vi "PauseSong.vi"(8 "error in (no error)":errorcluster, 10 "Message Queues in":T1, 11 "UI Refs in":T2) -> (0 "error out":errorcluster, 2 "Message Queues out":T1, 3 "UI Refs out":T2)   [LabVIEW 2015]
uses:
  Controls & Type Defs/UI Data.ctl
  support/Message Queue/All Message Queues.ctl
  support/Message Queue/Message Cluster.ctl
  support/Message Queue/Enqueue Message (Single).vi
  support/Message Queue/Message Queue.lvlib
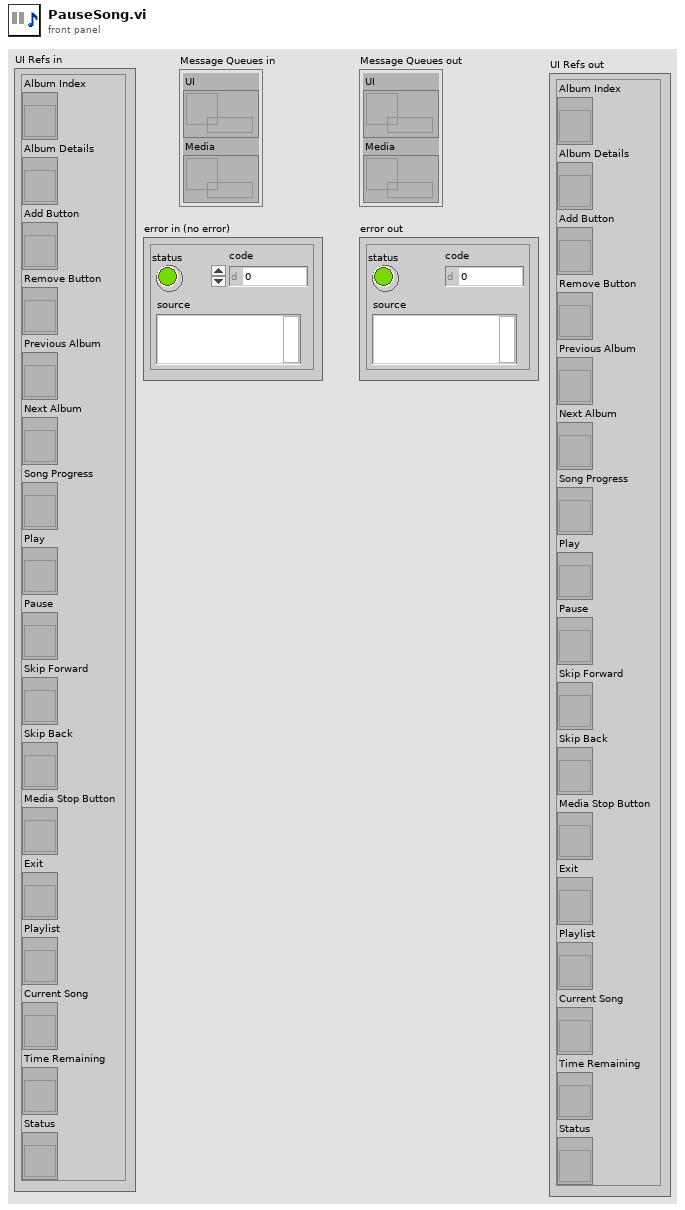
[diagram p1: front panel]
types:
  T1 = typedef "Message Queue.lvlib/All Message Queues.ctl" = cluster{"UI":refnum<queue>, "Media":refnum<queue>}
  T2 = typedef "UI Data.ctl" = cluster{"Album Index":refnum<vi>, "Album Details":refnum<vi>, "Add Button":refnum<vi>, "Remove Button":refnum<vi>, "Previous Album":refnum<vi>, "Next Album":refnum<vi>, "Song Progress":refnum<vi>, "Play":refnum<vi>, "Pause ":refnum<vi>, "Skip Forward":refnum<vi>, "Skip Back":refnum<vi>, "Media Stop Button":refnum<vi>, "Exit":refnum<vi>, "Playlist":refnum<vi>, "Current Song":refnum<vi>, "Time Remaining":refnum<vi>, "Status":refnum<vi>}
  T3 = enum8{"Enabled", "Disabled", "Disabled and Grayed Out"}
  T4 = typedef "Message Queue.lvlib/Message Cluster.ctl" = cluster{"Message":string, "Message Data":variant}
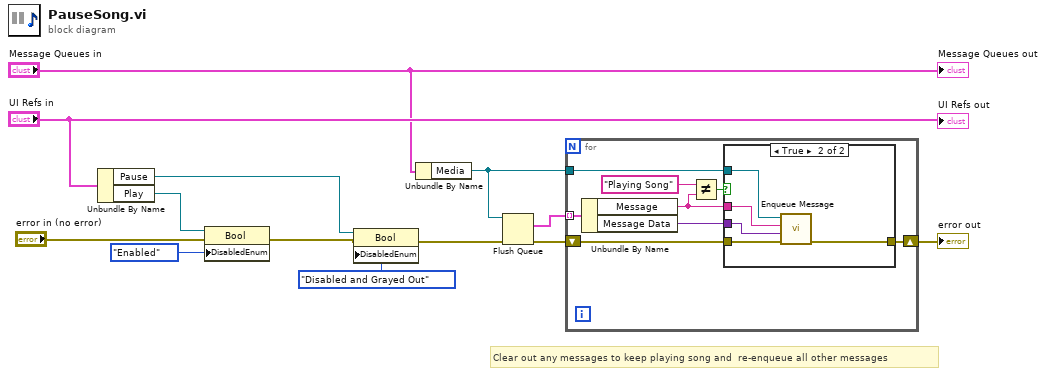
[diagram p0: block diagram]
diagram:
  # "Clear out any messages to keep playing song and  re-enqueue all other messages"
  n1 = Unbundle By Name("UI Refs in") -> ("Pause"=w8:refnum<vi>, "Play"=w9:refnum<vi>)
  n2 = property class="Bool"(reference=w9, error in="error in (no error)", "DisabledEnum"=T3."Enabled" ("Disabled")) -> (error out=w7:errorcluster)  [unwired: 1 out]
  n3 = property class="Bool"(reference=w8, error in=w7, "DisabledEnum"=T3."Disabled and Grayed Out" ("Disabled")) -> (error out=w3:errorcluster)  [unwired: 1 out]
  n4 = Unbundle By Name("Message Queues in") -> ("Media"=w2:refnum<queue>)
  n5 = Flush Queue(queue=w2, error in (no error)=w3) -> (remaining elements=w4:T4[], error out=w5:errorcluster)  [unwired: 1 out]
  n6 = for {
    shift-right: [w17] -> w1
    shift-left: w5 -> [w18]
    tunnel: w4 -> [w21] mode=indexing
    tunnel: w2 -> [w16]
    n7 = Unbundle By Name(w21) -> ("Message"=w14:string, "Message Data"=w15:variant)
    n8 = Not Equal?(x="Playing Song", y=w14) -> (x != y?=w19:bool)
    n9 = case shown="True" w19 {
      tunnel: w18 -> [w22 w27]
      tunnel: [w22 w26] -> w17
      tunnel: w16 -> [_ w25]
      tunnel: w15 -> [_ w24]
      tunnel: w14 -> [_ w23]
      frame False {
      }
      frame True {
        n10 = call-poly "Enqueue Message.vi"("error in (no error)"=w27, "Message Data"=w24, "Message"=w23, "Message Queue"=w25) -> ("error out"=w26:errorcluster)  [unwired: 6 in, 1 out]
      }
    }
  }
  "error out" <- w1
  "UI Refs out" <- "UI Refs in"
  "Message Queues out" <- "Message Queues in"
